vi "MathCad_Easy_Matrix_Set_2D.vi"(8 "error in (no error)":errorcluster, 9 "Data In":dbl[][](array[numeric]) format="%.2f", 10 "New Variable Name":string, 11 "Mathcad Reference":T1) -> (0 "error out":errorcluster, 3 "Mathcad Reference":T1)   [LabVIEW 2015]
doc: "Sets a 2-D matrix value in Mathcad. You can also use this VI to reset a variable that has already been set once. It is only dependent upon the variable name. The variables won't appear in the Mathcad worksheet, but are defined at the very beginning of the worksheet.\n\nInputs\nWrksht Ref--ActiveX Reference to Mathcad Worksheet Class\nNew Variable (String) -Name of Variable to Set\nData In (2D Array Double)- Data to set.\n \n\nOutputs\nWrksht Ref--ActiveX Reference to Mathcad Worksheet Class"
uses:
  Mathcad Reference.ctl
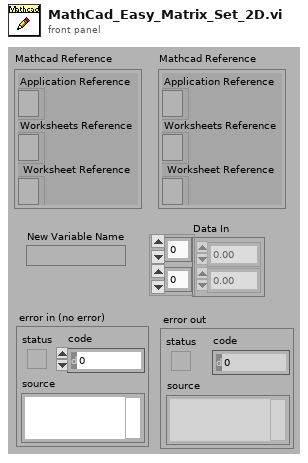
[diagram p1: front panel]
types:
  T1 = typedef "Mathcad Reference.ctl" = cluster{"Application Reference":refnum<k7>, "Worksheets Reference":refnum<k7>, " Worksheet Reference":refnum<k7>}
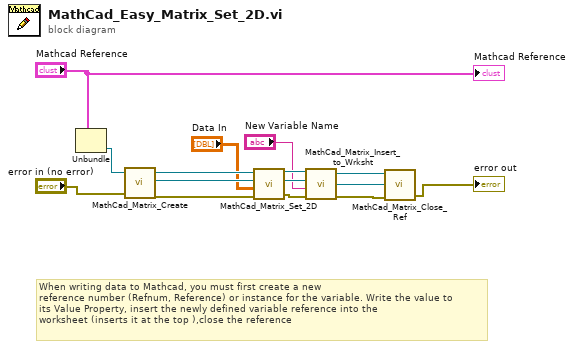
[diagram p0: block diagram]
diagram:
  # "When writing data to Mathcad, you must first create a new \nreference number (Refnum, Reference) or instance for the variable. Write the value to\nits Value Property, insert the newly defined variable reference into the\nworksheet (inserts it at the top ),close the reference"
  n1 = Unbundle("Mathcad Reference") -> ("Worksheet Reference"=w2:refnum<k7>)  [unwired: 2 out]
  n2 = call "MathCad_Matrix_Create.vi"("error in (no error)"="error in (no error)", "Worksheet Reference In"=w2) -> ("error out"=w12:errorcluster, "Mathcad.IMatrixValue Reference Out"=w13:refnum<k7>, "Worksheet Reference Out"=w14:refnum<k7>)  [unwired: 1 in]
  n3 = call "MathCad_Matrix_Set_2D.vi"("error in"=w12, "2D Array"="Data In", "Mathcad.IMatrixValue Refnum in"=w13, "Worksheet Reference In"=w14) -> ("error out"=w9:errorcluster, "Mathcad.IMatrixValue Refnum out"=w7:refnum<k7>, "Worksheet Reference Out"=w8:refnum<k7>)
  n4 = call "MathCad_Matrix_Insert_to_Wrksht.vi"("error out 2"=w9, "New Variable Name"="New Variable Name", "Mathcad.IMatrixValue Reference In"=w7, "Worksheet Reference In"=w8) -> ("error out"=w6:errorcluster, "Mathcad.IMatrixValue Reference Out"=w11:refnum<k7>, "Worksheet Reference Out"=w10:refnum<k7>)
  n5 = call "MathCad_Matrix_Close_Ref.vi"("error in"=w6, "Mathcad.IMatrixValue Reference"=w11, "IMathcadWorksheet Reference"=w10) -> ("error out"=→"error out":errorcluster)  [unwired: 2 in, 1 out]
  "Mathcad Reference" <- "Mathcad Reference"
